vi "실습 9-1.vi"() -> ()   [LabVIEW 2014]
uses:
  <vilib>/Analysis/NI_AALBase.lvlib
panel:
  out "웨이브폼 그래프":dbl[][](graph)
  out "텍스트":string
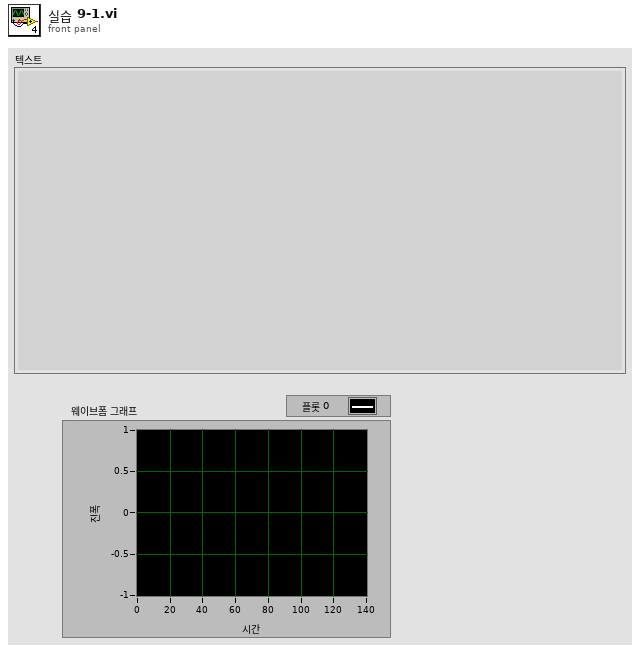
[diagram p1: front panel]
types:
  T1 = enum16{"open", "replace", "create", "open or create", "replace or create", "replace or create with confirmation"}
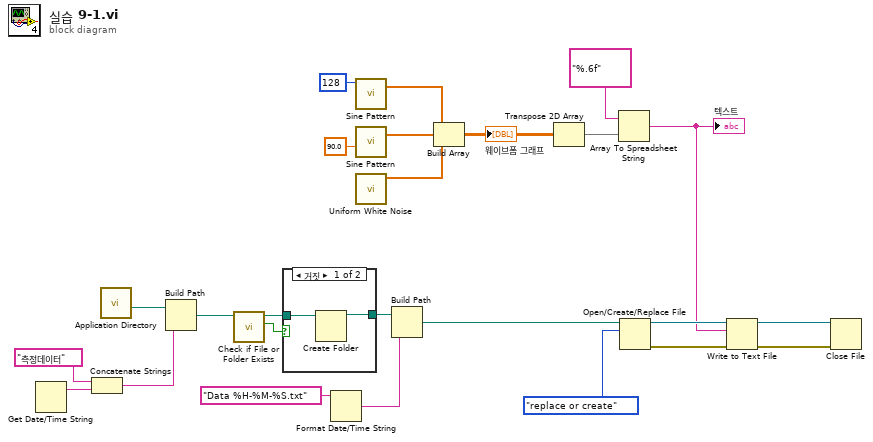
[diagram p0: block diagram]
diagram:
  n1 = Get Date/Time String() -> (date string=w25:string)  [unwired: 3 in, 1 out]
  n2 = Concatenate Strings("측정데이터" ("문자열"), w25) -> (w22:string)
  n3 = call <vilib>:"Application Directory.vi"() -> ("Application Directory"=w23:path)
  n4 = Build Path(base path=w23, name or relative path=w22) -> (appended path=w21:path)
  n5 = call <vilib>:"Check if File or Folder Exists.vi"("path"=w21) -> ("file or folder exists?"=w20:bool, "dup path"=w19:path)  [unwired: 8 in, 1 out]
  n6 = case shown="거짓" w20 {
    tunnel: w19 -> [w27 w28]
    tunnel: [w26 w28] -> w18
    frame False {
      n7 = Create Folder(path (use dialog)=w27) -> (created path=w26:path)  [unwired: 2 in, 2 out]
    }
    frame True {
    }
  }
  n8 = Format Date/Time String(time format string (%c)="Data %H-%M-%S.txt" ("시간 포맷 문자열 (%c)")) -> (date/time string=w17:string)  [unwired: 2 in]
  n9 = call <vilib>:"Sine Pattern.vi"("samples"=128) -> ("Sinusoidal Pattern"=w7:dbl[])  [unwired: 3 in, 1 out]
  n10 = call <vilib>:"Sine Pattern.vi"("phase(degrees)"=90.0) -> ("Sinusoidal Pattern"=w6:dbl[])  [unwired: 3 in, 1 out]
  n11 = call <vilib>:"Uniform White Noise.vi"() -> ("uniform white noise"=w5:dbl[])  [unwired: 10 in, 1 out]
  n12 = Build Path(base path=w18, name or relative path=w17) -> (appended path=w15:path)
  n13 = Build Array(w7, w6, w5) -> (w4:dbl[][])
  "웨이브폼 그래프" <- w4
  n14 = Transpose 2D Array(2D array=w4) -> (transposed array=w1:dbl[][])
  n15 = Array To Spreadsheet String(array=w1, 3:"%.6f" ("포맷 문자열")) -> (spreadsheet string=w3:string)  [unwired: 1 in]
  "텍스트" <- w3
  n16 = Open/Create/Replace File(file path (use dialog)=w15, operation (0:open)=T1."replace or create" ("동작(0:open)")) -> (refnum out=w13:refnum<file>, error out=w11:errorcluster)  [unwired: 4 in, 1 out]
  n17 = Write to Text File(file (use dialog)=w13, text=w3, error in=w11) -> (refnum out=w12:refnum<file>, error out=w10:errorcluster)  [unwired: 1 in, 1 out]
  n18 = Close File(refnum=w12, error in=w10) -> ()  [unwired: 2 out]
